vi "HackRF_Read_Complex.vi"(8 "error in (no error)":errorcluster, 10 "count":i32=1000, 11 "HackRF":T1) -> (0 "error out":errorcluster, 2 "Data":cdb[](array[numeric]), 3 "HackRF":T1)   [LabVIEW 2010]
uses:
  C:/Users/fl1ckje/Desktop/SDR/HackRF/labview/x64/NetHackrfx64.dll
  NetHackrfx64.dll
  HackRF_Ref.ctl
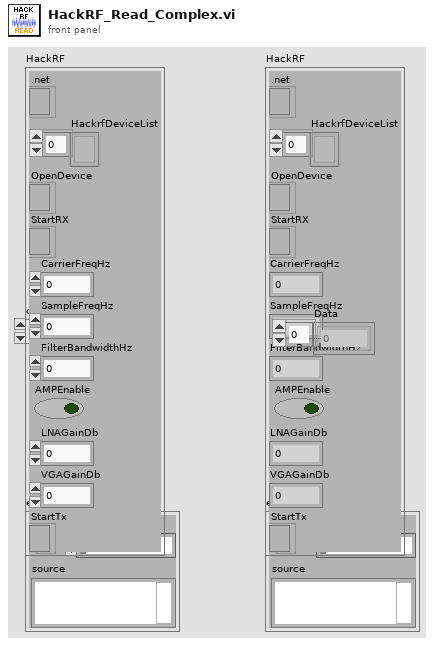
[diagram p1: front panel]
types:
  T1 = typedef "HackRF_Ref.ctl" = cluster{".net":refnum<k24>, "HackrfDeviceList":refnum<k24>[], "OpenDevice":refnum<k24>, "StartRX":refnum<k24>, "CarrierFreqHz":dbl, "SampleFreqHz":dbl, "FilterBandwidthHz":dbl, "AMPEnable":bool, "LNAGainDb":dbl, "VGAGainDb":dbl, "StartTx":refnum<k24>}
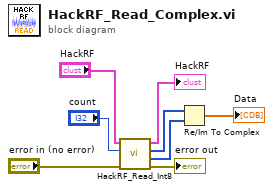
[diagram p0: block diagram]
diagram:
  n1 = call "HackRF_Read_Int8.vi"("error in (no error)"="error in (no error)", "count"="count", "HackRF"="HackRF") -> ("error out"=→"error out":errorcluster, "Q data"=w4:i8[], "I data"=w5:i8[], "HackRF"=→"HackRF":T1)  [unwired: 5 in]
  n2 = Re/Im To Complex(1:w4, 2:w5) -> (0:→"Data":cdb[])
